vi "PAN_GetCmdLineArgs.vi"() -> (6 "configpath":path, 14 "cmdlineapp":string)   [LabVIEW 2016]
panel:
  out "error out":errorcluster
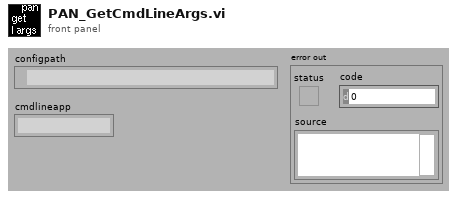
[diagram p1: front panel]
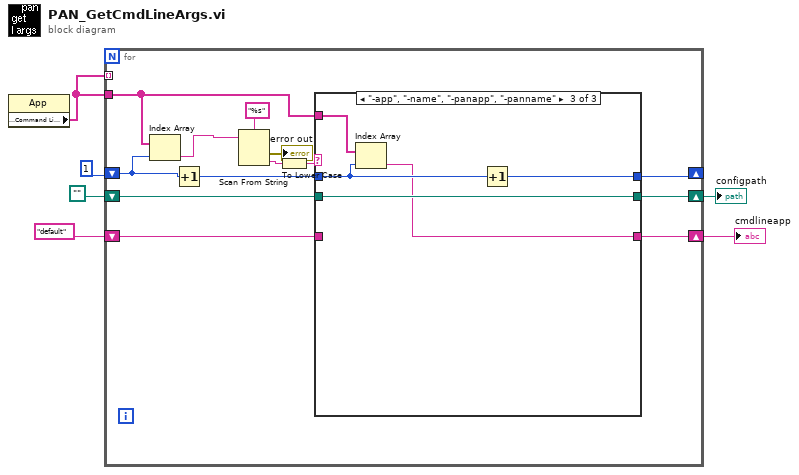
[diagram p0: block diagram]
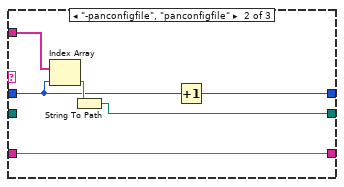
[diagram p3: hidden frame]
diagram:
  n1 = property class="App"() -> ("Application:Command Line Arguments"=w3:string[])  [unwired: 2 in, 2 out]
  n2 = for {
    shift-right: [w19] -> w5
    shift-left: path "" -> [w18]
    tunnel: w3 -> [w15]
    shift-right: [w13] -> _
    shift-left: 1 ("index") -> [w16]
    tunnel: w3 -> [_] mode=indexing
    shift-right: [w7] -> w2
    shift-left: "default" ("element") -> [w8]
    n3 = Index Array(array=w15, index=w16) -> (element=w14:string)
    n4 = Increment(x=w16) -> (x+1=w17:i32)
    n5 = Scan From String(format string="%s", input string=w14) -> (error out=→"error out":errorcluster, output 1=w10:string)  [unwired: 2 in, 3 out]
    n6 = To Lower Case(string=w10) -> (all lower case string=w11:string)
    n7 = case shown="\"-app\", \"-name\", \"-panapp\", \"-panname\"" w11 {
      tunnel: [w22 w28 w30] -> w19
      tunnel: w18 -> [w22 _ w30]
      tunnel: w15 -> [_ w27 w33]
      tunnel: w17 -> [w21 w25 w32]
      tunnel: [w21 w24 w31] -> w13
      tunnel: w8 -> [w20 w23 _]
      tunnel: [w20 w23 w29] -> w7
      frame Default {
      }
      frame "-panconfigfile", "panconfigfile" {
        n8 = Index Array(array=w27, index=w25) -> (element=w26:string)
        n9 = String To Path(string=w26) -> (path=w28:path)
        n10 = Increment(x=w25) -> (x+1=w24:i32)
      }
      frame "-app", "-name", "-panapp", "-panname" {
        n11 = Index Array(array=w33, index=w32) -> (element=w29:string)
        n12 = Increment(x=w32) -> (x+1=w31:i32)
      }
    }
  }
  "configpath" <- w5
  "cmdlineapp" <- w2
